vi "LabVIEW GUI - hysteresis.vi"() -> ()   [LabVIEW 2021]
uses:
  <vilib>/Instr/_visa.llb/VISA Configure Serial Port (Instr).vi
panel:
  out "Thermometer":dbl(slide) scale=0.0..40.0
  out "LED":bool
  out "Buffer":string
  out "Waveform Chart":cluster{"Thermometer":dbl, dbl, dbl, i32}(graph)
  in  "stop":bool
  in  "Arduino COM Port":refnum<visa-resource-name>="COM3"
  # "Thermistor-based Thermostat with hysteresys"
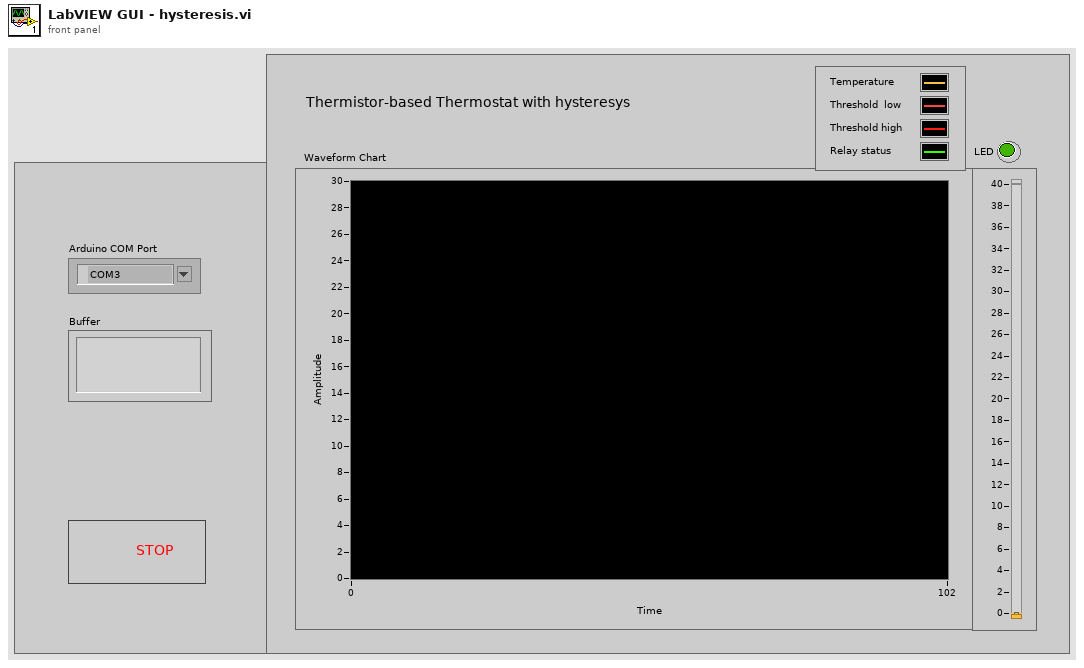
[diagram p1: front panel]
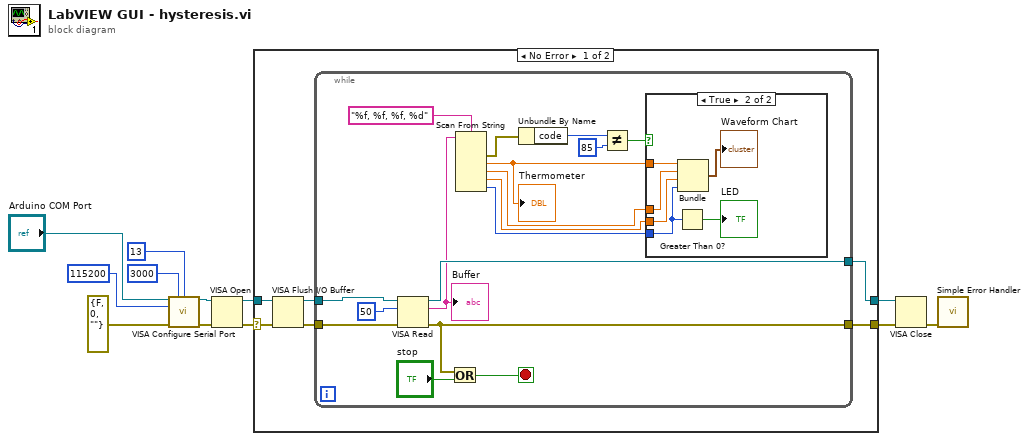
[diagram p0: block diagram]
diagram:
  n1 = call-poly "VISA Configure Serial Port"("VISA resource name"="Arduino COM Port", "timeout (10sec)"=u32 3000, "termination char\n(0xA = '\\n' = LF)"=u8 13 ("termination char\n(0xA = '\\n' = LF)"), "baud rate (9600)"=u32 115200, "error in (no error)"=errorcluster {"status"=FALSE, "code"=0, "source"=""}) -> ("VISA resource name out"=w7:refnum<visa-resource-name>, "error out"=w8:errorcluster)  [unwired: 9 in]
  n2 = VISA Open(error in (no error)=w8, VISA resource name=w7) -> (VISA resource name=w6:refnum<visa-resource-name>, error out=w5:errorcluster)  [unwired: 3 in]
  n3 = case shown="No Error" w5 {
    selector: w5 -> [w15 w42]
    tunnel: w6 -> [w16 w43]
    tunnel: [w18 w42] -> w3
    tunnel: [w17 w43] -> w2
    frame No Error {
      n4 = VISA Flush I/O Buffer(VISA resource name=w16, error in (no error)=w15) -> (VISA resource name out=w14:refnum<visa-resource-name>, error out=w13:errorcluster)  [unwired: 1 in]
      n5 = while {
        tunnel: w14 -> [w34]
        tunnel: [w33] -> w17
        tunnel: w13 -> [w35]
        tunnel: [w21] -> w18
        stop <- w19 stop-if-true
        n6 = VISA Read(VISA resource name=w34, byte count=u32 50, error in (no error)=w35) -> (VISA resource name out=w33:refnum<visa-resource-name>, read buffer=w25:string, error out=w21:errorcluster)  [unwired: 1 out]
        "Buffer" <- w25
        n7 = Or(x=w21, y="stop") -> (x .or. y?=w19:bool)
        n8 = Scan From String(format string="%f, %f, %f, %d", input string=w25) -> (error out=w29:errorcluster, output 1=w24:dbl, output 2=w30:dbl, output 3=w23:dbl, output 4=w22:i32)  [unwired: 6 in, 2 out]
        "Thermometer" <- w24
        n9 = Unbundle By Name(w29) -> ("code"=w28:i32)
        n10 = Not Equal?(x=w28, y=85) -> (x != y?=w26:bool)
        n11 = case shown="True" w26 {
          tunnel: w24 -> [_ w41]
          tunnel: w30 -> [_ w40]
          tunnel: w23 -> [_ w37]
          tunnel: w22 -> [_ w36]
          frame False {
          }
          frame True {
            n12 = Greater Than 0?(x=w36) -> (x > 0?=→"LED":bool)
            n13 = Bundle("Thermometer"=w41, w40, w37, w36) -> (→"Waveform Chart":cluster{"Thermometer":dbl, dbl, dbl, i32})  [unwired: 1 in]
          }
        }
      }
    }
    frame Error {
    }
  }
  n14 = VISA Close(VISA resource name=w2, error in (no error)=w3) -> (error out=w1:errorcluster)
  n15 = call <vilib>:"Simple Error Handler.vi"("error in (no error)"=w1) -> ()  [unwired: 4 in, 5 out]
